vi "Neutral_Agilent_E3631A_TriggerSet_20151208.vi"(4 "Triggered Current Limit":dbl=1.0 format="%.2g", 5 "Initial Current Limit":dbl=1.0 format="%.3g", 6 "Triggered Voltage Level":dbl=5.0 format="%.3g", 7 "Initial Voltage Level":dbl=1.0 format="%.3g", 9 "Trigger Delay (s)":dbl min=0.0 max=3600.0 step=1.0 format="%.2f", 10 "Channel":i32(ring)=1 items=["+6V"=1, "+24V"=2, "-24V"=3], 11 "VISA resource name":refnum<visa-resource-name>) -> ()   [LabVIEW 2015]
doc: "This example demonstrates the triggering functionality of the power supply. Initial and triggered voltage and limit settings are configured. The Send Software Trigger VI is used to trigger the instrument."
uses:
  Agilent Driver/Agilent E363X Series.lvlib
panel:
  # "Initial Voltage Settings"
  # "Triggered Settings"
  # "(c) 2008 National Instruments.  ALL RIGHTS RESERVED."
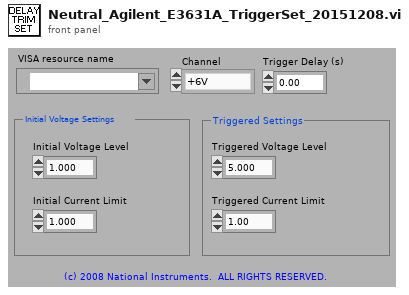
[diagram p1: front panel]
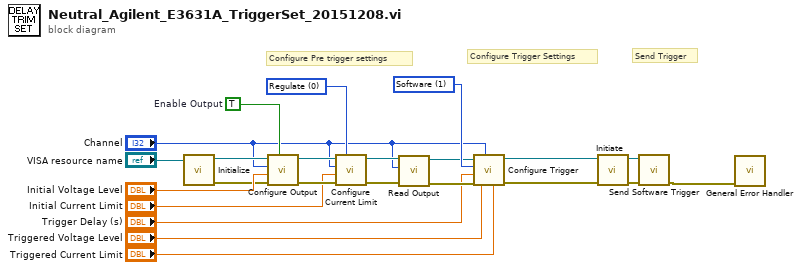
[diagram p0: block diagram]
diagram:
  w13 = u16 0 items=["Regulate", "Trip"] ("Behavior (0: Regulate)")
  w19 = u16 1 items=["Immediate", "Software"] ("Trigger Source (0: Immediate)")
  w23 = TRUE  # Enable Output
  # "Configure Pre trigger settings"
  # "Send Trigger"
  # "Configure Trigger Settings"
  n1 = call "Initialize.vi"("VISA resource name"="VISA resource name") -> ("error out"=w16:errorcluster, "VISA resource name out"=w17:refnum<visa-resource-name>)  [unwired: 9 in]
  n2 = call "Configure Output.vi"("Enable Output (T: Enable)"=w23, "error in (no error)"=w16, "Voltage Level (0.0 V)"="Initial Voltage Level", "Channel (1: Channel 1)"="Channel", "VISA resource name"=w17) -> ("error out"=w14:errorcluster, "VISA resource name out"=w15:refnum<visa-resource-name>)  [unwired: 5 in]
  n3 = call "Configure Current Limit.vi"("Behavior (0: Regulate)"=w13, "error in (no error)"=w14, "Current Limit (0.0 A)"="Initial Current Limit", "Channel (1: Channel 1)"="Channel", "VISA resource name"=w15) -> ("error out"=w5:errorcluster, "VISA resource name out"=w6:refnum<visa-resource-name>)  [unwired: 5 in]
  n4 = call "Read Output.vi"("error in (no error)"=w5, "Channel (1: Channel 1)"="Channel", "VISA resource name"=w6) -> ("error out"=w4:errorcluster, "VISA resource name out"=w3:refnum<visa-resource-name>)  [unwired: 5 in, 2 out]
  n5 = call "Configure Trigger.vi"("Triggered Current Limit (0.0 A)"="Triggered Current Limit", "Triggered Voltage Level (0.0 V)"="Triggered Voltage Level", "Channel (1: Channel 1)"="Channel", "error in (no error)"=w4, "Trigger Delay (0 sec)"="Trigger Delay (s)", "Trigger Source (0: Immediate)"=w19, "VISA resource name"=w3) -> ("error out"=w20:errorcluster, "VISA resource name out"=w21:refnum<visa-resource-name>)  [unwired: 3 in]
  n6 = call "Initiate.vi"("error in (no error)"=w20, "VISA resource name"=w21) -> ("error out"=w8:errorcluster, "VISA resource name out"=w9:refnum<visa-resource-name>)  [unwired: 8 in]
  n7 = call "Send Software Trigger.vi"("error in (no error)"=w8, "VISA resource name"=w9) -> ("error out"=w7:errorcluster)  [unwired: 8 in, 1 out]
  n8 = call <vilib>:"General Error Handler.vi"("error in (no error)"=w7) -> ()  [unwired: 10 in, 5 out]
